vi "Controller Test Bench (16).vi"() -> ()   [LabVIEW 2022 SP3]
uses:
  WhiteNoise.ctl
  <vilib>/sound2/lvsound2.llb/Sound Data Format.ctl
  <vilib>/Utility/error.llb/DialogType.ctl
  <vilib>/sound2/lvsound2.llb/Sampling Mode.ctl
  <vilib>/Platform/TimedLoop/XDataNode/timing_clust.ctl
  <vilib>/Platform/TimedLoop/XDataNode/nitl_modes.ctl
  <vilib>/Platform/TimedLoop/XDataNode/wakeup.ctl
  <vilib>/sound2/lvsound2.llb/Sound File Refnum.ctl
  <vilib>/Analysis/4window.llb/windowTd.ctl
  <vilib>/DAQmx/write.llb/DAQmx Write (Analog 1D Wfm NChan NSamp).vi
  <vilib>/DAQmx/read.llb/DAQmx Read (Analog 1D Wfm NChan NSamp).vi
  <vilib>/DAQmx/create/channels.llb/DAQmx Create Channel (AI-Acceleration-Accelerometer).vi
  <vilib>/DAQmx/configure/timing.llb/DAQmx Timing (Sample Clock).vi
  <vilib>/Platform/TimedLoop/scheduler/LVUserAPI/_suppVIs/Create_1kHz_TSource.vi
  <vilib>/DAQmx/create/channels.llb/DAQmx Create Channel (AO-Voltage-Basic).vi
  <vilib>/sound2/lvsound2.llb/Sound File Info (path).vi
  <vilib>/sound2/lvsound2.llb/Sound File Read Open.vi
  <vilib>/sound2/lvsound2.llb/Sound File Read (DBL).vi
  <vilib>/DAQmx/miscellaneous.llb/DAQmx Fill In Error Info.vi
  <vilib>/sound2/lvsound2.llb/Sound Output Set Volume (Single).vi
  <vilib>/sound2/lvsound2.llb/Sound Output Write (DBL).vi
  <vilib>/addons/control/pid/pid.llb/PID (DBL Array).vi
  <vilib>/sound2/lvsound2.llb/Sound Output Write (DBL Single).vi
  <vilib>/DAQmx/configure/task.llb/DAQmx Configure Logging (TDMS).vi
  <vilib>/measure/maspectr.llb/FFT Spectrum (Mag-Phase) for N Chan.vi
  <vilib>/platform/TimedLoop/XDataNode/XDataNode.xnode
  <vilib>/measure/NI_MAPro.lvlib
  <resource>/objmgr/daqmx.rc
  <vilib>/Analysis/NI_AALPro.lvlib
  <vilib>/measure/NI_MABase.lvlib
  <vilib>/addons/control/pid/NI_PID_pid.lvlib
  <vilib>/Platform/TimedLoop/XDataNode/XDNodeRunTimeDep.lvlib
panel:
  in  "Time Out (s)":dbl=1000.0
  out "Elapsed Time":i32 caption="Elapsed Time (s)" format="%.2f"
  in  "Time Out (s)":dbl=1000.0
  out "Active Controller Output":dbl[](graph)
  out "Elapsed Time":i32 caption="Elapsed Time (s)" format="%.2f"
  in  "Acquisition\nPeriod(ms)":dbl=41.2
  out "Accel.1":waveform(dbl)[](graph)
  out "Excitation Output":waveform(dbl)[](graph)
  in  "Output Noise":bool=TRUE
  in  "?":T1(tab)=enum."Harmonic"
  in  "Cluster 3":T2={"Path txt/csv File"=path "C:/Users/LAV-UFSC-2023/Documents/LAV-TCC/Dados-Experimentos/acc_time/Previous Data/handlebar_acc1_run2.txt", "Delimiter"=".", "Separator"="\\t", "Offset (lines)"=21.0}
  in  "Gain":i32
  in  "Stop 3":bool
  in  "Gain":i32
  in  "Cluster 4":T4={"Seed"=0.0, "Iterator"=1.0, "Path Sound File"=path "C:/Users/LAV-UFSC-2023/Documents/LAV-TCC/Dados-Experimentos/Dados Empíricos/Uni-cheio.wav", "number of samples/ch (-1: all)"=-1}
  in  "Stop 2":bool
  in  "Cluster":T5={"Seed"=0.0, "Standard Deviation"=0.2, "Reset"=FALSE, "Iterator"=1.0, "Seed"=-1, "Stop 4"=FALSE, "Lower Cut-Off 2"=5.0, "Upper Cut-Off 2"=350.0} {"Upper Cut-Off 2" min=5.0 max=350.0 step=10.0; "Lower Cut-Off 2" min=5.0 max=350.0 step=10.0; "Standard Deviation" min=0.001 max=1.5 step=0.05 format="%0.2p"}
  in  "Cluster 2":T6={"Iterator"=1.0, "Waveform Type"=0, "Frequency"=10.0, "Amplitude"=0.25, "Stop 4"=FALSE} {"Frequency" min=5.0 max=350.0 step=10.0 format="%0.2p"; "Waveform Type" items=["Sine Wave", "Triangle Wave", "Square Wave", "Sawtooth Wave"]; "Amplitude" min=0.001 max=0.3 step=0.05 format="%0.2p"}
  in  "Active Control":bool
  in  "Tab Control":T7(tab)
  out "dt out (s)":dbl format="%.3f"
  in  "setpoint":dbl[](array[numeric])=[0.0] format="%.2f"
  in  "PID gains":T8(array[cluster])=[{"proportional gain (Kc)"=1.0, "integral time (Ti, min)"=0.01, "derivative time (Td, min)"=0.0}] {"derivative time (Td, min)" step=0.0025 format="%.3e"; "integral time (Ti, min)" step=0.0025 format="%.3e"; "proportional gain (Kc)" step=0.0025 format="%.3e"}
  in  "dt (s)":dbl=-1.0 format="%.3f"
  in  "output range":cluster{"output high":dbl, "output low":dbl}[](array[cluster])=[{"output high"=100.0, "output low"=-100.0}] {"output low" format="%.2f"; "output high" format="%.2f"}
  in  "Upper Cut-Off":dbl=130.0
  in  "Lower Cut-Off":dbl=70.0
  in  "Setpoint":dbl
  in  "Gain":dbl min=0.0 step=0.01
  out "Output Signal":dynamicdata(graph)
  in  "Upper Cut-Off":dbl=400.0
  in  "Lower Cut-Off":dbl=100.0
  out "Accel.2":waveform(dbl)[](graph)
  in  "Log Raw Data":bool
  out "Mag 2":cluster{"f0":dbl, "df":dbl, "magnitude":dbl[]}[](graph)
  in  "Show FFT":bool=TRUE
  in  "Log FFT":bool
  in  "Start Reading":bool=TRUE
  in  "Stop":bool
  # "Active Controller"
  # "Main\nSwitch"
  # "Output Noise"
  # "RAW - Accel. 1"
  # "Data Acquisition"
  # "FFT - Amplitude (dB)"
  # "RAW - Accel. 2"
  # "Runtime"
  # "Pre-Set"
  # "Runtime"
  # "Pre-Set"
  # "Runtime"
  # "Filter"
  # "Runtime"
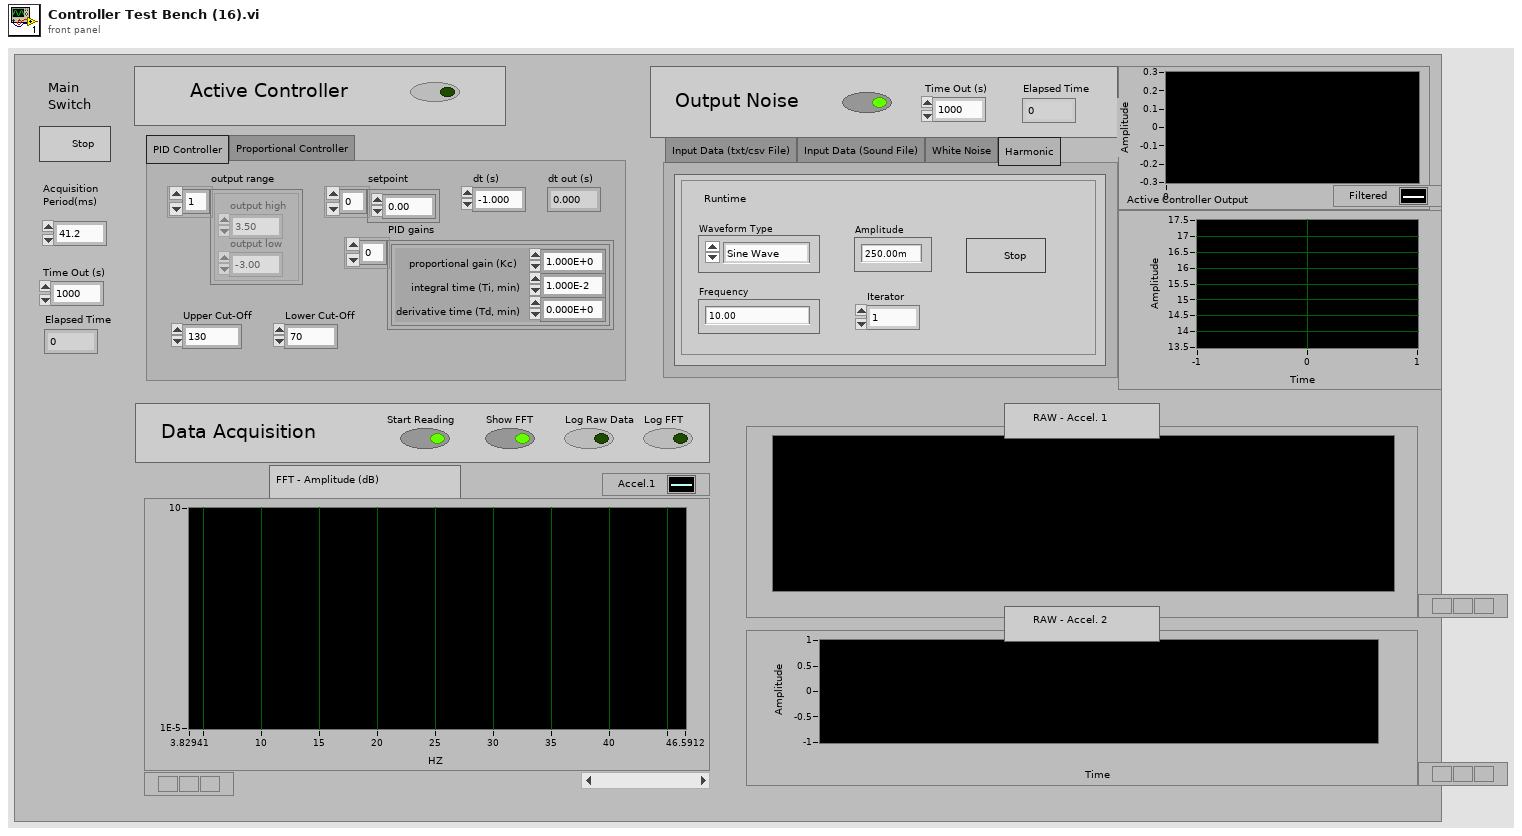
[diagram p1: front panel]
types:
  T1 = enum32{"Input Data (txt/csv File)", "Input Data (Sound File)", "White Noise", "Harmonic"}
  T2 = cluster{"Path txt/csv File":path, "Delimiter":string, "Separator":string, "Offset (lines)":dbl}
  T3 = typedef "WhiteNoise.ctl" = dbl
  T4 = cluster{"Seed":T3, "Iterator":dbl, "Path Sound File":path, "number of samples/ch (-1: all)":i32}
  T5 = cluster{"Seed":T3, "Standard Deviation":dbl, "Reset":bool, "Iterator":dbl, "Seed":i8, "Stop 4":bool, "Lower Cut-Off 2":dbl, "Upper Cut-Off 2":dbl}
  T6 = cluster{"Iterator":dbl, "Waveform Type":u16, "Frequency":dbl, "Amplitude":dbl, "Stop 4":bool}
  T7 = enum32{"PID Controller", "Proportional Controller"}
  T8 = cluster{"proportional gain (Kc)":dbl, "integral time (Ti, min)":dbl, "derivative time (Td, min)":dbl}[]
  T9 = typedef "Sampling Mode.ctl" = i32
  T10 = typedef "DialogType.ctl" = u16
  T11 = typedef "Sound Data Format.ctl" = cluster{"sample rate (S/s)":dbl, "number of channels":i32, "bits per sample":i32}
  T12 = typedef "Sound File Refnum.ctl" = refnum<file>
  T13 = typedef "XDNodeRunTimeDep.lvlib/timing_clust.ctl" = cluster{"Expected End [f-1]":u64, "Actual End [f-1]":u64, "Finished Late? [f-1]":bool, "Expected End [i-1]":u64, "Actual End [i-1]":u64, "Finished Late? [i-1]":bool, "Expected Start [i]":u64, "Actual Start [i]":u64, "Expected Start [f]":u64, "Actual Start [f]":u64, "Source Name":string, "Structure Name":string, "Period":i64, "Deadline":i64, "Offset":i64, "Start":i64, "Priority":i32, "Timeout":i32, "Mode":T14, "Wakeup Reason":T15, "Error":errorcluster, "Source Type":string, "Secondary Source Type":string, "Global End Time":u64, "Global Start Time":u64, "Frame Duration":u64, "Iteration Duration":u64, "Assigned CPU":i32, "I/O Scan Engine Mode":u32}
  T14 = typedef "XDNodeRunTimeDep.lvlib/nitl_modes.ctl" = enum32{"No Change", "Process missed periods, maintain original phase", "Discard missed periods, maintain original phase", "Process missed periods, ignore original phase", "Discard missed periods, ignore original phase"}
  T15 = typedef "XDNodeRunTimeDep.lvlib/wakeup.ctl" = enum32{"Normal", "Aborted", "Asynchronous wakeup", "Timing source error", "Timed loop error", "Timeout"}
  T16 = typedef "Sound Output Task ID.ctl" = u32
  T17 = typedef "NI_AALPro.lvlib/windowTd.ctl" = u32
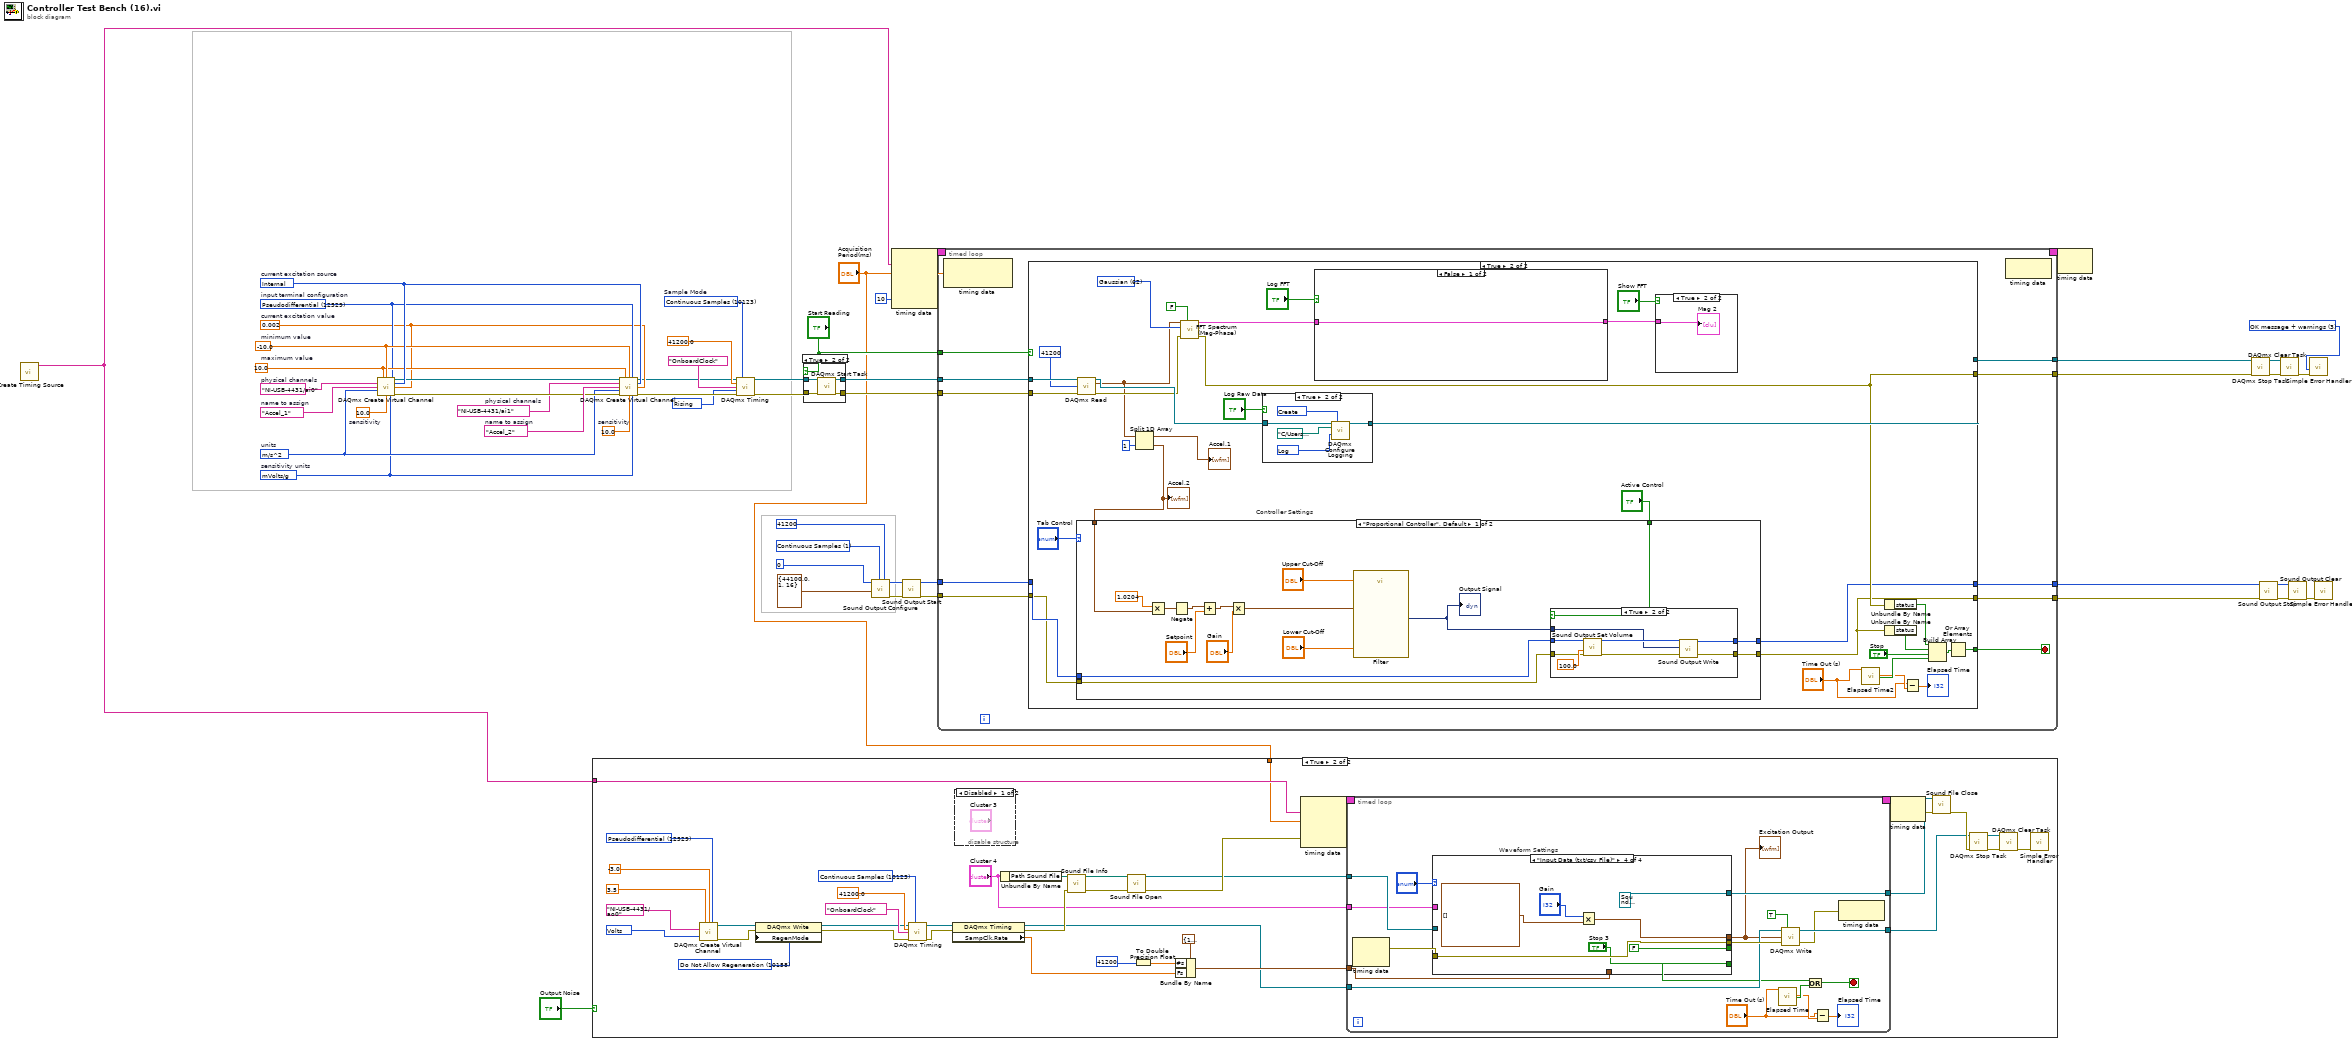
[diagram p0: block diagram]
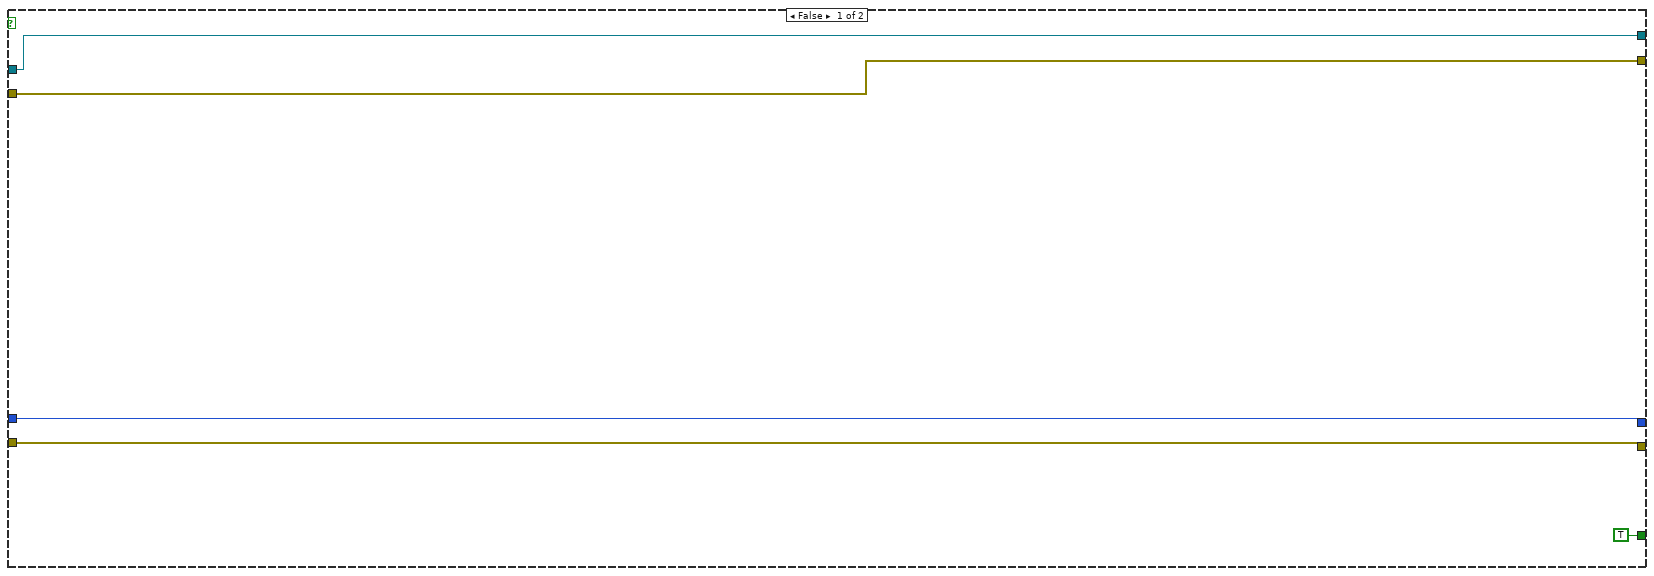
[diagram p2: hidden frame]
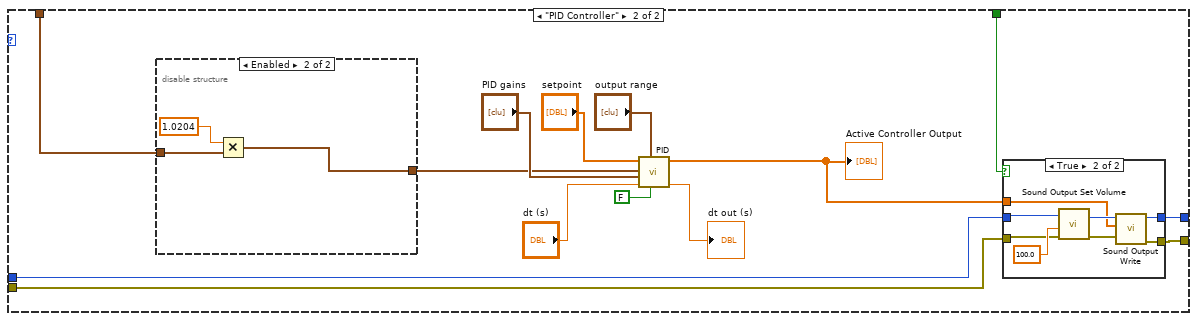
[diagram p4: hidden frame]
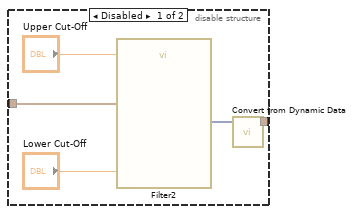
[diagram p5: hidden frame]
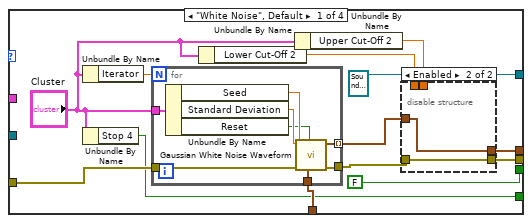
[diagram p12: hidden frame]
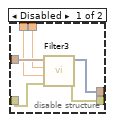
[diagram p13: hidden frame]
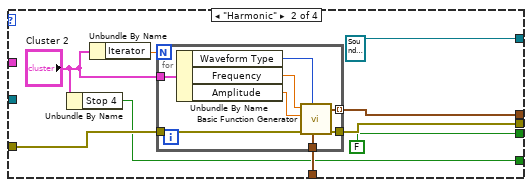
[diagram p14: hidden frame]
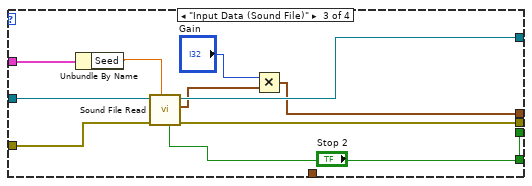
[diagram p15: hidden frame]
diagram:
  w3 = 10280 items=["Rising"=10280, "Falling"=10171] ("active edge")
  w5 = 12509 items=["mVolts/g"=12509, "Volts/g"=12510]  # sensitivity units
  w40 = 10.0  # sensitivity
  w4 = 0.002  # current excitation value
  w34 = 10200 items=["Internal"=10200, "External"=10167, "None"=10230]  # current excitation source
  w26 = tag "NI-USB-4431/ai0"  # physical channels
  w39 = 10123 items=["Finite Samples"=10178, "Continuous Samples"=10123, "Hardware Timed Single Point"=12522]  # Sample Mode
  w29 = 12529 items=["default"=-1, "RSE"=10083, "NRSE"=10078, "Differential"=10106, "Pseudodifferential"=12529]  # input terminal configuration
  w32 = -10.0  # minimum value
  w31 = 10.0  # maximum value
  w41 = "Accel_1"  # name to assign
  w30 = 12470 items=["g"=10186, "m/s^2"=12470, "in/s^2"=12471, "From Custom Scale"=10065]  # units
  w42 = 10.0  # sensitivity
  w27 = tag "NI-USB-4431/ai1"  # physical channels
  w36 = "Accel_2"  # name to assign
  w43 = T9 1 items=["Finite Samples", "Continuous Samples"] ("sample mode")
  w44 = T10 3 items=["no dialog", "OK message", "continue or stop message", "OK message + warnings", "continue/stop + warnings"] ("type of dialog (OK msg:1)")
  n1 = call-poly <vilib>:"Create Timing Source.vi"() -> ("name (out)"=w15:string)  [unwired: 10 in, 1 out]
  n2 = call-poly <vilib>:"DAQmx Create Virtual Channel.vi"("maximum value"=w31, "minimum value"=w32, "input terminal configuration"=w29, "physical channels"=w26, "current excitation source"=w34, "name to assign"=w41, "current excitation value"=w4, "units"=w30, "sensitivity"=w40, "sensitivity units"=w5) -> ("task out"=w28:refnum<k21>, "error out"=w35:errorcluster)  [unwired: 4 in]
  n3 = case shown="True" "Output Noise" {
    tunnel: w15 -> [_ w62]
    tunnel: "Acquisition\nPeriod(ms)" -> [_ w52]
    frame False {
    }
    frame True {
      w78 = 10123 items=["Finite Samples"=10178, "Continuous Samples"=10123, "Hardware Timed Single Point"=12522] ("sample mode")
      w82 = 10158 items=["Allow Regeneration"=10097, "Do Not Allow Regeneration"=10158] ("RegenMode")
      w88 = 12529 items=["Default"=-1, "RSE"=10083, "Differential"=10106, "Pseudodifferential"=12529] ("output terminal configuration")
      w86 = 10348 items=["Volts"=10348, "From Custom Scale"=10065] ("units")
      n4 = call-poly <vilib>:"DAQmx Create Virtual Channel.vi"("maximum value"=3.5, "minimum value"=-3.0, "output terminal configuration"=w88, "physical channels"=tag "NI-USB-4431/ao0", "units"=w86) -> ("task out"=w81:refnum<k21>, "error out"=w83:errorcluster)  [unwired: 9 in]
      n5 = property class="DAQmx Write"(reference=w81, error in=w83, "RegenMode"=w82) -> (reference out=w79:refnum<k21>, error out=w80:errorcluster)
      n6 = call-poly <vilib>:"DAQmx Timing.vi"("task/channels in"=w79, "sample mode"=w78, "rate"=41200.0 ("Sample Rate"), "source"=tag "OnboardClock" ("Sample Clock Source"), "error in"=w80) -> ("task out"=w74:refnum<k21>, "error out"=w73:errorcluster)  [unwired: 9 in]
      n7 = property class="DAQmx Timing"(reference=w74, error in=w73) -> (reference out=w57:refnum<k21>, error out=w67:errorcluster, "SampClk.Rate"=w75:dbl)
      n8 = disable-structure shown="Disabled" {
        frame Disabled {
        }
        frame Enabled {
        }
      }
      n9 = Unbundle By Name("Cluster 4") -> ("Path Sound File"=w55:path)
      n10 = call-poly <vilib>:"Sound File Info.vi"("error in (no error)"=w67, "path"=w55) -> ("error out"=w69:errorcluster, "path out"=w68:path)  [unwired: 6 in, 2 out]
      n11 = call-poly <vilib>:"Sound File Open.vi"("error in (no error)"=w69, "path"=w68) -> ("error out"=w63:errorcluster, "sound file refnum"=w61:T12)  [unwired: 8 in]
      n12 = To Double Precision Float(number=41200) -> (double precision float=w76:dbl)
      n13 = Bundle By Name(cluster=cluster{"Fs":dbl, "#s":dbl} {"Fs"=1000.0, "#s"=1000.0} ("sampling info"), "#s"=w76, "Fs"=w75) -> (w58:cluster{"Fs":dbl, "#s":dbl})
      n14 = node-c288(w62, w52, w63) -> (w65:T13)  [unwired: 1 in]
      n15 = timed-loop {
        timing: w65 -> [_]
        timing-out: [_] -> w64
        tunnel: w61 -> [w104]
        tunnel: [w103] -> w60
        tunnel: [w102] -> w59
        tunnel: w58 -> [w101]
        tunnel: w57 -> [w100]
        tunnel: "Cluster 4" -> [w99]
        stop <- w97 stop-if-true
        # "Waveform Settings"
        n16 = node-c288() -> (w105:errorcluster)  [unwired: 1 in, 1 out]
        n17 = case shown="\"Input Data (txt/csv File)\"" "?" {
          tunnel: w101 -> [w121 w144 _ _]
          tunnel: w105 -> [w119 w146 w165 w170]
          tunnel: [w112 w143 w164 w170] -> w107
          tunnel: [w114 w145 w160 w166] -> w98
          tunnel: w104 -> [_ _ w163 _]
          tunnel: [FALSE FALSE w162 FALSE ("end of file?")] -> _
          tunnel: [T12 refnum ("sound file refnum out") T12 refnum ("sound file refnum out") w161 T12 refnum ("sound file refnum out")] -> w103
          tunnel: w99 -> [_ _ w157 _]
          tunnel: [w116 w138 "Stop 2" "Stop 3"] -> w96
          frame "White Noise", Default {
            n18 = Unbundle By Name("Cluster") -> ("Iterator"=w120:dbl)
            n19 = Unbundle By Name("Cluster") -> ("Stop 4"=w116:bool)
            n20 = for {
              N: w120 -> [_]
              tunnel: w119 -> [w137]
              tunnel: w121 -> [w136]
              tunnel: [w135] -> w113
              tunnel: "Cluster" -> [w134]
              tunnel: [w133] -> w115 mode=indexing
              n21 = Unbundle By Name(w134) -> ("Seed"=w132:T3, "Standard Deviation"=w131:dbl, "Reset"=w130:bool)
              n22 = call <vilib>:"Gaussian White Noise Waveform.vi"("sampling info"=w136, "reset signal"=w130, "error in (no error)"=w137, "seed"=w132, "standard deviation"=w131) -> ("error out"=w135:errorcluster, "signal out"=w133:waveform(dbl))  [unwired: 5 in]
            }
            n23 = Unbundle By Name("Cluster") -> ("Lower Cut-Off 2"=w110:dbl)
            n24 = Unbundle By Name("Cluster") -> ("Upper Cut-Off 2"=w109:dbl)
            n25 = disable-structure shown="Enabled" {
              disable-tunnel: w115 -> [w127 w129]
              disable-tunnel: [w126 w129] -> w114
              disable-tunnel: w113 -> [w125 w128]
              disable-tunnel: [w124 w128] -> w112
              disable-tunnel: w110 -> [w123 _]
              disable-tunnel: w109 -> [w122 _]
              frame Disabled {
                n26 = call "Filter3"("error in (no error)"=w125, "Lower Cut-Off"=w123, "Upper Cut-Off"=w122, "Signal"=w127) -> ("error out"=w124:errorcluster, "Filtered Signal"=w126:dynamicdata)  [unwired: 6 in]
              }
              frame Enabled {
              }
            }
          }
          frame "Harmonic" {
            n27 = Unbundle By Name("Cluster 2") -> ("Stop 4"=w138:bool)
            n28 = Unbundle By Name("Cluster 2") -> ("Iterator"=w142:dbl)
            n29 = for {
              N: w142 -> [_]
              tunnel: w146 -> [w154]
              tunnel: w144 -> [w153]
              tunnel: [w152] -> w143
              tunnel: "Cluster 2" -> [w151]
              tunnel: [w147] -> w145 mode=indexing
              n30 = Unbundle By Name(w151) -> ("Waveform Type"=w150:u16, "Frequency"=w149:dbl, "Amplitude"=w148:dbl)
              n31 = call <vilib>:"Basic Function Generator.vi"("sampling info"=w153, "signal type"=w150, "error in (no error)"=w154, "amplitude"=w148, "frequency"=w149) -> ("error out"=w152:errorcluster, "signal out"=w147:waveform(dbl))  [unwired: 4 in, 1 out]
            }
          }
          frame "Input Data (Sound File)" {
            n32 = Unbundle By Name(w157) -> ("Seed"=w158:T3)
            n33 = call-poly <vilib>:"Sound File Read.vi"("number of samples/ch (-1: all)"=w158, "error in (no error)"=w165, "sound file refnum"=w163) -> ("error out"=w164:errorcluster, "data"=w159:waveform(dbl)[], "sound file refnum out"=w161:T12, "end of file?"=w162:bool)  [unwired: 4 in, 1 out]
            n34 = Multiply(x="Gain", y=w159) -> (x*y=w160:waveform(dbl)[])
          }
          frame "Input Data (txt/csv File)" {
            n35 = Multiply(x="Gain", y=waveform(dbl)[] []) -> (x*y=w166:waveform(dbl)[])
          }
        }
        "Excitation Output" <- w98
        n36 = call "Elapsed Time"("Time Target (s)"="Time Out (s)") -> ("Elapsed Time (s)"=w92:dbl, "Time has Elapsed"=w93:bool)  [unwired: 11 in, 6 out]
        n37 = call-poly <vilib>:"DAQmx Write.vi"("task/channels in"=w100, "auto start"=TRUE, "data"=w98, "error in"=w107) -> ("task out"=w102:refnum<k21>, "error out"=w95:errorcluster)  [unwired: 9 in, 1 out]
        n38 = Or(x=w96, y=w93) -> (x .or. y?=w97:bool)
        n39 = Subtract(x="Time Out (s)", y=w92) -> (x-y=→"Elapsed Time":dbl)
        n40 = node-c288(w95) -> ()  [unwired: 1 out]
      }
      n41 = node-c288(w64) -> (w53:errorcluster)
      n42 = call <vilib>:"Sound File Close.vi"("error in (no error)"=w53, "sound file refnum"=w60) -> ("error out"=w66:errorcluster)  [unwired: 9 in]
      n43 = call <vilib>:"DAQmx Stop Task.vi"("task/channels in"=w59, "error in"=w66) -> ("task out"=w72:refnum<k21>, "error out"=w71:errorcluster)  [unwired: 12 in]
      n44 = call <vilib>:"DAQmx Clear Task.vi"("task in"=w72, "error in"=w71) -> ("error out"=w70:errorcluster)  [unwired: 13 in]
      n45 = call <vilib>:"Simple Error Handler.vi"("error in (no error)"=w70) -> ()  [unwired: 4 in, 5 out]
    }
  }
  n46 = call-poly <vilib>:"DAQmx Create Virtual Channel.vi"("task in"=w28, "maximum value"=w31, "minimum value"=w32, "input terminal configuration"=w29, "physical channels"=w27, "current excitation source"=w34, "name to assign"=w36, "current excitation value"=w4, "units"=w30, "error in"=w35, "sensitivity"=w42, "sensitivity units"=w5) -> ("task out"=w1:refnum<k21>, "error out"=w33:errorcluster)  [unwired: 2 in]
  n47 = call-poly <vilib>:"DAQmx Timing.vi"("task/channels in"=w1, "sample mode"=w39, "rate"=41200.0 ("Sample Rate"), "source"=tag "OnboardClock" ("Sample Clock Source"), "active edge"=w3, "error in"=w33) -> ("task out"=w24:refnum<k21>, "error out"=w25:errorcluster)  [unwired: 8 in]
  n48 = case shown="True" "Start Reading" {
    tunnel: w25 -> [w185 w190]
    tunnel: w24 -> [w186 w189]
    tunnel: [w186 w188] -> w11
    tunnel: [w185 w187] -> w12
    frame False {
    }
    frame True {
      n49 = call <vilib>:"DAQmx Start Task.vi"("task/channels in"=w189, "error in"=w190) -> ("task out"=w188:refnum<k21>, "error out"=w187:errorcluster)  [unwired: 12 in]
    }
  }
  n50 = call <vilib>:"Sound Output Configure.vi"("number of samples/ch"=41200 ("Number of Samples/ch"), "sample mode"=w43, "sound format"=T11 {"sample rate (S/s)"=44100.0, "number of channels"=1, "bits per sample"=16} ("Sound Format"), "device ID"=u32 0 ("Device ID")) -> ("error out"=w20:errorcluster, "task ID"=w19:T16)  [unwired: 6 in]
  n51 = node-c288(w15, "Acquisition\nPeriod(ms)", i64 10 ("Offset")) -> (w17:T13)  [unwired: 2 in]
  n52 = call <vilib>:"Sound Output Start.vi"("error in (no error)"=w20, "task ID"=w19) -> ("error out"=w13:errorcluster, "task ID out"=w14:T16)  [unwired: 8 in]
  n53 = timed-loop {
    timing: w17 -> [_]
    timing-out: [_] -> w16
    tunnel: "Start Reading" -> [w200]
    tunnel: w14 -> [w199]
    tunnel: w13 -> [w198]
    tunnel: w12 -> [w197]
    tunnel: w11 -> [w196]
    tunnel: [w195] -> w10
    tunnel: [w194] -> w9
    tunnel: [w193] -> w8
    tunnel: [w192] -> w7
    stop <- w191 stop-if-true
    n54 = node-c288() -> ()  [unwired: 1 in, 2 out]
    n55 = case shown="True" w200 {
      tunnel: w196 -> [w205 w238]
      tunnel: w197 -> [w204 w237]
      tunnel: [w205 w234] -> w194
      tunnel: [w204 w224] -> w195
      tunnel: w199 -> [w202 w218]
      tunnel: w198 -> [w203 w217]
      tunnel: [w202 w214] -> w193
      tunnel: [w203 w215] -> w192
      tunnel: [TRUE w211] -> w191
      frame False {
      }
      frame True {
        w223 = T17 62 items=["Rectangle"=0, "Hanning"=1, "Hamming"=2, "Blackman-Harris"=3, "Exact Blackman"=4, "Blackman"=5, "Flat Top"=6, "4 Term B-Harris "=7, "7 Term B-Harris"=8, "Low Sidelobe"=9, "Blackman Nuttall"=11, "Triangle"=30, "Bartlett-Hanning"=31, "Bohman"=32, "Parzen"=33, "Welch"=34, "Kaiser"=60, "Dolph-Chebyshev"=61, "Gaussian"=62] ("window")
        # "Controller Settings"
        n56 = call-poly <vilib>:"DAQmx Read.vi"("task/channels in"=w238, "number of samples per channel"=41200, "error in"=w237) -> ("task out"=w235:refnum<k21>, "data"=w213:waveform(dbl)[], "error out"=w225:errorcluster)  [unwired: 10 in]
        n57 = Split 1D Array(array=w213, index=1) -> (first subarray=→"Accel.1":waveform(dbl)[], second subarray=w206:waveform(dbl)[])
        "Accel.2" <- w206
        n58 = case shown="\"Proportional Controller\", Default" "Tab Control" {
          tunnel: w206 -> [w240 w265]
          tunnel: w218 -> [w247 w273]
          tunnel: w217 -> [w248 w272]
          tunnel: "Active Control" -> [w246 w271]
          tunnel: [w250 w270] -> w214
          tunnel: [w249 w269] -> w215
          frame "Proportional Controller", Default {
            n59 = Multiply(x=1.0204, y=w240) -> (x*y=w241:waveform(dbl)[])
            n60 = Negate(x=w241) -> (-x=w253:waveform(dbl)[])
            n61 = Add(x=w253, y="Setpoint") -> (x+y=w252:waveform(dbl)[])
            n62 = Multiply(x=w252, y="Gain") -> (x*y=w245:waveform(dbl)[])
            n63 = call "Filter"("Lower Cut-Off"="Lower Cut-Off", "Upper Cut-Off"="Upper Cut-Off", "Signal"=w245) -> ("Filtered Signal"=w244:dynamicdata)  [unwired: 7 in, 1 out]
            "Output Signal" <- w244
            n64 = case shown="True" w246 {
              tunnel: w248 -> [w256 w262]
              tunnel: [w256 w259] -> w249
              tunnel: w247 -> [w255 w263]
              tunnel: [w255 w258] -> w250
              tunnel: w244 -> [_ w257]
              frame False {
              }
              frame True {
                n65 = call-poly <vilib>:"Sound Output Set Volume.vi"("error in (no error)"=w262, "volume"=100.0, "task ID"=w263) -> ("error out"=w260:errorcluster, "task ID out"=w261:T16)  [unwired: 7 in]
                n66 = call-poly <vilib>:"Sound Output Write.vi"("error in (no error)"=w260, "data"=w257, "task ID"=w261) -> ("error out"=w259:errorcluster, "task ID out"=w258:T16)  [unwired: 7 in]
              }
            }
          }
          frame "PID Controller" {
            n67 = disable-structure shown="Enabled" {
              disable-tunnel: [w280 w284] -> w266
              disable-tunnel: w265 -> [w279 w285]
              frame Disabled {
                n68 = call "Filter2"("Lower Cut-Off"="Lower Cut-Off", "Upper Cut-Off"="Upper Cut-Off", "Signal"=w279) -> ("Filtered Signal"=w281:dynamicdata)  [unwired: 7 in, 1 out]
                n69 = call "Convert from Dynamic Data"("Dynamic Data Type"=w281) -> ("Array"=w280:dbl[])  [unwired: 3 in]
              }
              frame Enabled {
                n70 = Multiply(x=1.0204, y=w285) -> (x*y=w284:waveform(dbl)[])
              }
            }
            n71 = call-poly <vilib>:"PID.vi"("reinitialize? (F)"=FALSE, "output range"="output range", "dt (s)"="dt (s)", "PID gains"="PID gains", "process variable"=w266, "setpoint"="setpoint") -> ("dt out (s)"=→"dt out (s)":dbl, "output"=w267:dbl[])  [unwired: 4 in]
            "Active Controller Output" <- w267
            n72 = case shown="True" w271 {
              tunnel: w272 -> [w288 w294]
              tunnel: [w288 w291] -> w269
              tunnel: w273 -> [w287 w295]
              tunnel: [w287 w290] -> w270
              tunnel: w267 -> [_ w289]
              frame False {
              }
              frame True {
                n73 = call-poly <vilib>:"Sound Output Set Volume.vi"("error in (no error)"=w294, "volume"=100.0, "task ID"=w295) -> ("error out"=w292:errorcluster, "task ID out"=w293:T16)  [unwired: 7 in]
                n74 = call-poly <vilib>:"Sound Output Write.vi"("error in (no error)"=w292, "data"=w289, "task ID"=w293) -> ("error out"=w291:errorcluster, "task ID out"=w290:T16)  [unwired: 7 in]
              }
            }
          }
        }
        n75 = call-poly <vilib>:"FFT Spectrum (Mag-Phase).vi"("restart averaging (F)"=FALSE, "error in (no error)"=w225, "window"=w223, "time signals"=w213) -> ("error out"=w224:errorcluster, "magnitudes"=w229:cluster{"f0":dbl, "df":dbl, "magnitude":dbl[]}[])  [unwired: 3 in, 3 out]
        n76 = case shown="True" "Log Raw Data" {
          tunnel: w235 -> [w300 w302]
          tunnel: [w300 w301] -> w234
          frame False {
          }
          frame True {
            w303 = 15848 items=["Open"=10437, "Open or Create"=15846, "Create or Replace"=15847, "Create"=15848] ("operation")
            w304 = 15844 items=["Off"=10231, "Log"=15844, "Log and Read"=15842] ("logging mode")
            n77 = call-poly <vilib>:"DAQmx Configure Logging.vi"("task/channels in"=w302, "operation"=w303, "file path"=path "C:/Users/LAV-UFSC/Documents/LAV - TCC", "logging mode"=w304) -> ("task out"=w301:refnum<k21>)  [unwired: 10 in, 1 out]
          }
        }
        n78 = case shown="False" "Log FFT" {
          tunnel: w229 -> [w297 w298]
          tunnel: [w297 w298] -> w228
          frame False {
          }
          frame True {
          }
        }
        n79 = case shown="True" "Show FFT" {
          tunnel: w228 -> [_ w299]
          frame False {
          }
          frame True {
            "Mag 2" <- w299
          }
        }
        n80 = call "Elapsed Time2"("Time Target (s)"="Time Out (s)") -> ("Elapsed Time (s)"=w208:dbl, "Time has Elapsed"=w210:bool)  [unwired: 11 in, 6 out]
        n81 = Unbundle By Name(w224) -> ("status"=w221:bool)
        n82 = Unbundle By Name(w215) -> ("status"=w227:bool)
        n83 = Subtract(x="Time Out (s)", y=w208) -> (x-y=→"Elapsed Time":dbl)
        n84 = Build Array(w221, w227, "Stop", w210) -> (w232:bool[])
        n85 = Or Array Elements(Boolean array=w232) -> (logical OR=w211:bool)
      }
    }
    n86 = node-c288() -> ()  [unwired: 1 in, 1 out]
  }
  n87 = node-c288(w16) -> ()  [unwired: 1 out]
  n88 = call <vilib>:"DAQmx Stop Task.vi"("task/channels in"=w9, "error in"=w10) -> ("task out"=w47:refnum<k21>, "error out"=w46:errorcluster)  [unwired: 12 in]
  n89 = call <vilib>:"Sound Output Stop.vi"("error in (no error)"=w7, "task ID"=w8) -> ("error out"=w23:errorcluster, "task ID out"=w22:T16)  [unwired: 8 in]
  n90 = call <vilib>:"DAQmx Clear Task.vi"("task in"=w47, "error in"=w46) -> ("error out"=w48:errorcluster)  [unwired: 13 in]
  n91 = call <vilib>:"Sound Output Clear.vi"("error in (no error)"=w23, "task ID"=w22) -> ("error out"=w21:errorcluster)  [unwired: 9 in]
  n92 = call <vilib>:"Simple Error Handler.vi"("type of dialog (OK msg:1)"=w44, "error in (no error)"=w48) -> ()  [unwired: 3 in, 5 out]
  n93 = call <vilib>:"Simple Error Handler.vi"("error in (no error)"=w21) -> ()  [unwired: 4 in, 5 out]
